vi "Test CR5 Data Read.vi"() -> ()   [LabVIEW 2015]
uses:
  Data/CR5 Data.lvclass
  <vilib>/Utility/miscctls.llb/LVDateTimeRec.ctl
  Data/CR5 Data.lvclass/CR5 Data.ctl
  Data/Accessors/Write Balance.vi
  Data/Accessors/Write Tamb.vi
  Data/Accessors/Write Tmirror.vi
  Data/Accessors/Write flag.vi
  Data/Accessors/Write PWM.vi
  Data/Accessors/Write mirror flag.vi
  Data/Accessors/Write Tboard.vi
  Reusable/Data/Write measTime.vi
panel:
  out "error out":errorcluster
  out "reference out":refnum<class "CR5 Data.lvclass">
  in  "string":string
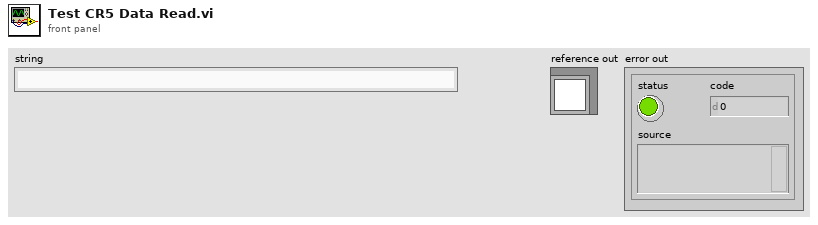
[diagram p1: front panel]
types:
  T1 = typedef "LVDateTimeRec.ctl" = cluster{"fractional second":dbl, "second":i32, "minute":i32, "hour":i32, "day of month":i32, "month":i32, "year":i32, "day of week":i32, "day of year":i32, "DST":i32}
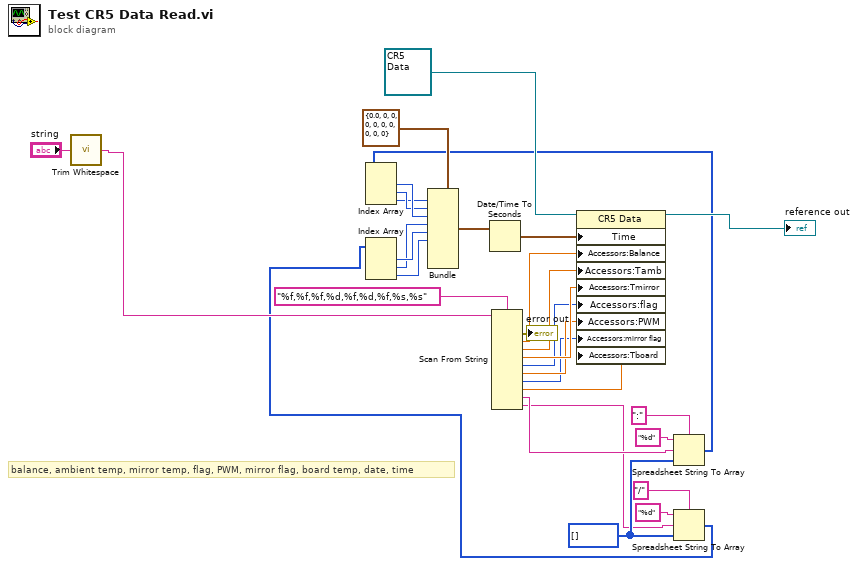
[diagram p0: block diagram]
diagram:
  w9 = i32[] []
  # "balance, ambient temp, mirror temp, flag, PWM, mirror flag, board temp, date, time"
  n1 = call <vilib>:"Trim Whitespace.vi"("string"="string") -> ("trimmed string"=w21:string)  [unwired: 1 in]
  n2 = Scan From String(format string="%f,%f,%f,%d,%f,%d,%f,%s,%s", input string=w21) -> (error out=→"error out":errorcluster, output 1=w17:dbl, output 2=w16:dbl, output 3=w15:dbl, output 4=w14:i32, output 5=w13:dbl, output 6=w12:i32, output 7=w11:dbl, output 8=w4:string, output 9=w3:string)  [unwired: 11 in, 2 out]
  n3 = Spreadsheet String To Array(delimiter (Tab)=":", format string="%d", spreadsheet string=w4, array type (2D Dbl)=w9) -> (array=w2:i32[])
  n4 = Index Array(array=w2) -> (element #1=w24:i32, element #2=w23:i32, element #3=w22:i32)  [unwired: 3 in]
  n5 = Spreadsheet String To Array(delimiter (Tab)="/", format string="%d", spreadsheet string=w3, array type (2D Dbl)=w9) -> (array=w1:i32[])
  n6 = Index Array(array=w1) -> (element #1=w27:i32, element #2=w26:i32, element #3=w25:i32)  [unwired: 3 in]
  n7 = Bundle(cluster=T1 {"fractional second"=0.0, "second"=0, "minute"=0, "hour"=0, "day of month"=0, "month"=0, "year"=0, "day of week"=0, "day of year"=0, "DST"=0} ("date time rec"), "second"=w22, "minute"=w23, "hour"=w24, "day of month"=w26, "month"=w27, "year"=w25) -> (w30:T1)  [unwired: 4 in]
  n8 = Date/Time To Seconds(2:w30) -> (0:w28:timestamp)  [unwired: 1 in]
  n9 = property class="CR5 Data"(reference=refnum<class "CR5 Data.lvclass"> refnum ("CR5 Data"), "Time"=w28, "Accessors:Balance"=w17, "Accessors:Tamb"=w16, "Accessors:Tmirror"=w15, "Accessors:flag"=w14, "Accessors:PWM"=w13, "Accessors:mirror flag"=w12, "Accessors:Tboard"=w11) -> (reference out=→"reference out":refnum<class "CR5 Data.lvclass">)  [unwired: 1 in, 1 out]
